vi "clearbuf.vi"(1 "error in (no error)":errorcluster) -> (0 "error out":errorcluster)   [LabVIEW 2017]
doc: "Clears any charcters in buffer"
uses:
  m_globals.vi
panel:
  in  "Case Constant\n(See Context Help)":bool
  in  "ACK":string="\u0006\u0000"
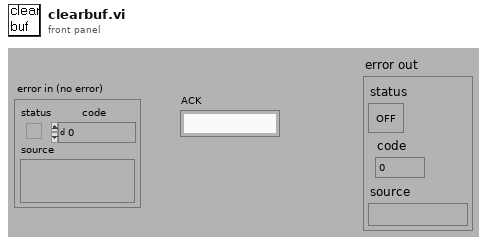
[diagram p1: front panel]
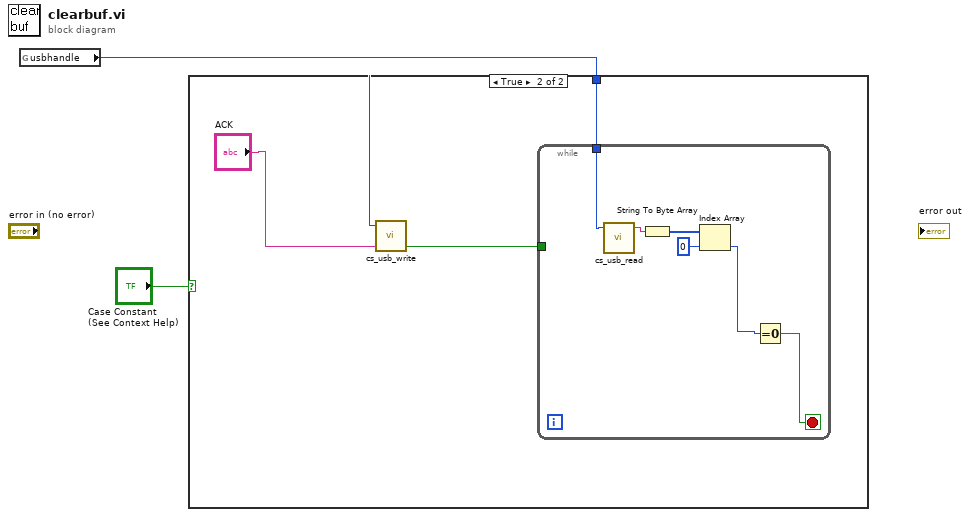
[diagram p0: block diagram]
diagram:
  n1 = global read "m_globals.vi" "usbhandle"() -> (w2:i32)
  n2 = case shown="True" "Case Constant\n(See Context Help)" {
    tunnel: w2 -> [_ w5]
    frame False {
    }
    frame True {
      n3 = call "cs_usb_write.vi"("string to send"="ACK", "handle"=w5) -> ("Error"=w3:bool)  [unwired: 3 in]
      n4 = while {
        tunnel: w5 -> [w11]
        tunnel: w3 -> [_]
        stop <- w6 stop-if-true
        n5 = call "cs_usb_read.vi"("handle"=w11) -> ("string"=w10:string)  [unwired: 3 in, 1 out]
        n6 = String To Byte Array(string=w10) -> (unsigned byte array=w9:u8[])
        n7 = Index Array(array=w9, index=0) -> (element=w7:u8)
        n8 = Equal To 0?(x=w7) -> (x = 0?=w6:bool)
      }
    }
  }
